vi "Write Error.vi"(8 "error in (no error)":errorcluster, 10 "Error":errorcluster, 11 "LogRecord in":refnum<class "LogRecord.lvclass">) -> (0 "error out":errorcluster, 3 "LogRecord out":refnum<class "LogRecord.lvclass">)   [LabVIEW 2024, in "hse-logger.lvlib" / "LogRecord.lvclass"]
doc: "____\nHAMPEL SOFTWARE ENGINEERING v2.2.2 (2025-01-16 15:41)"
uses:
  <vilib>/Hampel Software Engineering/HSE Logger/LogRecord/LogRecord.lvclass
  <vilib>/Hampel Software Engineering/HSE Logger/LogRecord/LogRecord.lvclass/LogRecord.ctl
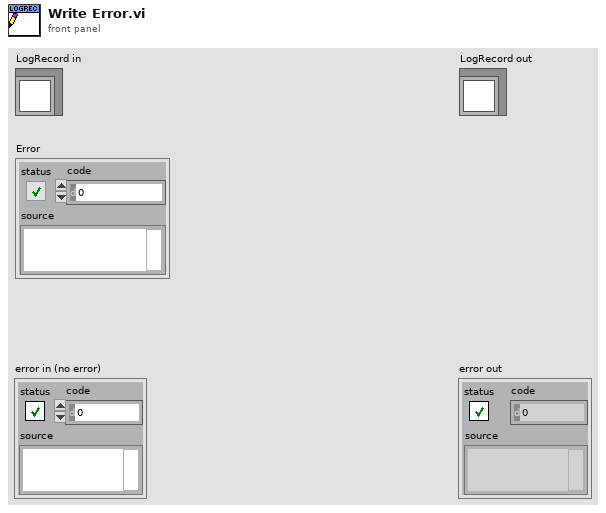
[diagram p1: front panel]
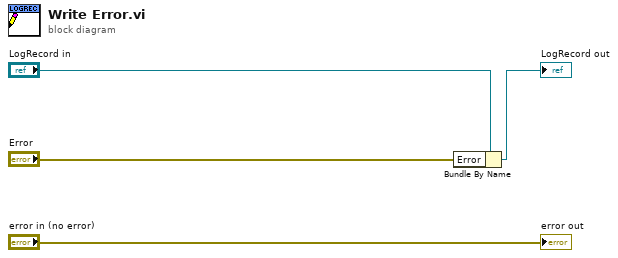
[diagram p0: block diagram]
diagram:
  n1 = Bundle By Name(cluster="LogRecord in", "Error"="Error") -> (→"LogRecord out":refnum<class "LogRecord.lvclass">)
  "error out" <- "error in (no error)"
